vi "fio.vi"() -> ()   [LabVIEW 2015]
uses:
  <vilib>/Utility/file.llb/Read Delimited Spreadsheet (DBL).vi
panel:
  out "Waveform Graph":waveform(dbl)(graph)
  out "subarray":dbl[](array[numeric])
  out "appended path":path
  out "all rows":dbl[][](array[numeric])
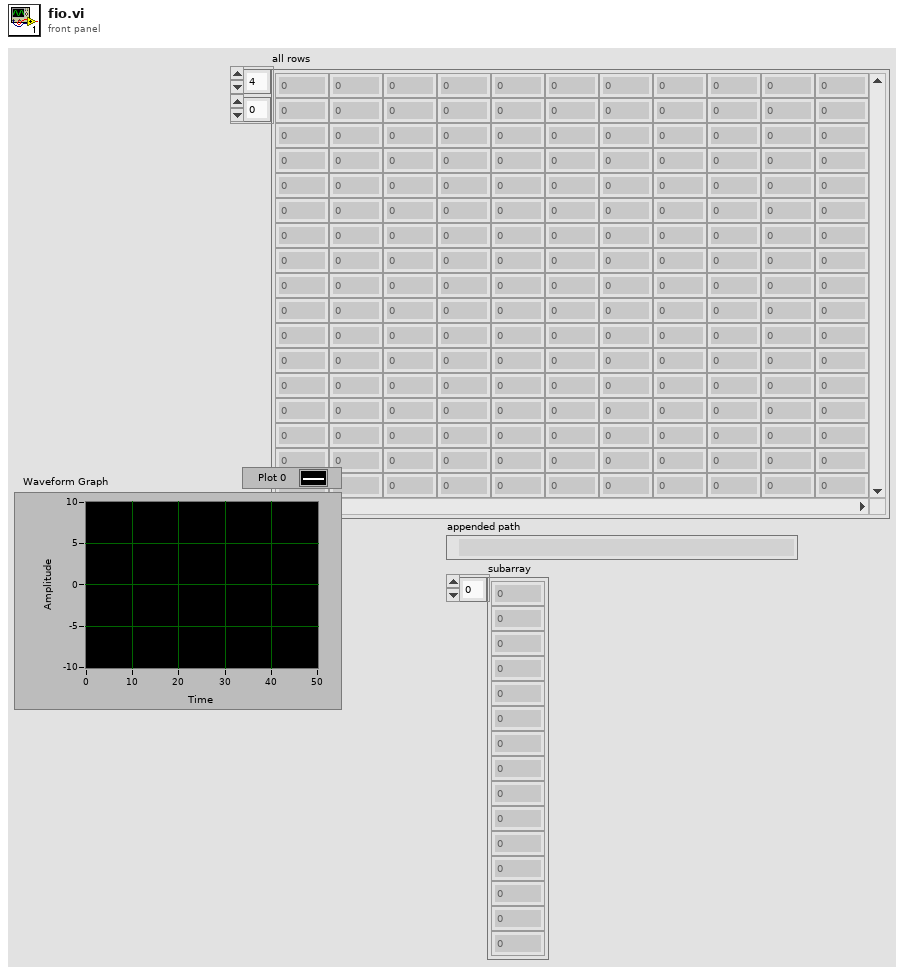
[diagram p1: front panel]
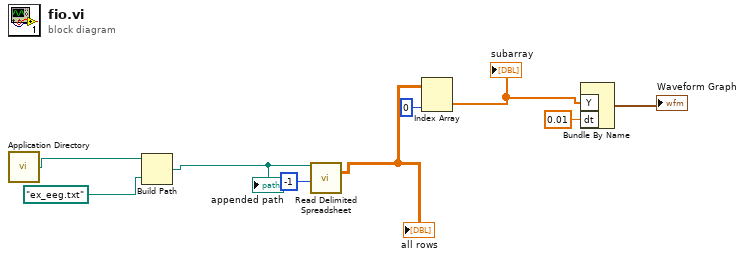
[diagram p0: block diagram]
diagram:
  n1 = call <vilib>:"Application Directory.vi"() -> ("Application Directory"=w6:path)
  n2 = Build Path(base path=w6, name or relative path=path "ex_eeg.txt" ("file path (dialog if empty)")) -> (appended path=w7:path)
  "appended path" <- w7
  n3 = call-poly <vilib>:"Read Delimited Spreadsheet.vi"("file path (dialog if empty)"=w7, "number of rows (all:-1)"=-1) -> ("all rows"=w5:dbl[][])  [unwired: 8 in, 5 out]
  "all rows" <- w5
  n4 = Index Array(array=w5, index (col)=0 ("disabled index (col)")) -> (element=w3:dbl[])  [unwired: 1 in]
  "subarray" <- w3
  n5 = Bundle By Name("Y"=w3, "dt"=0.01) -> (→"Waveform Graph":waveform(dbl))  [unwired: 1 in]
